vi "Modified Open URL in Default Browser core.vi"(4 "error in (no error)":errorcluster, 6 "Force IE? (F)":bool, 7 "url":string) -> (0 "error out":errorcluster, 3 "duplicate url":string)   [LabVIEW 2011]
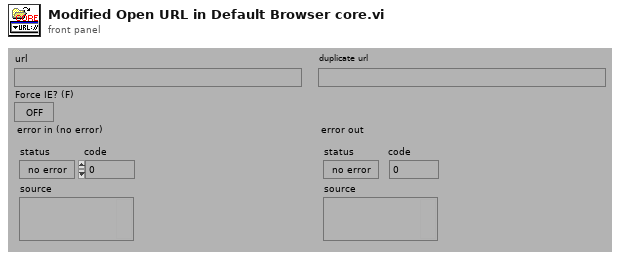
[diagram p1: front panel]
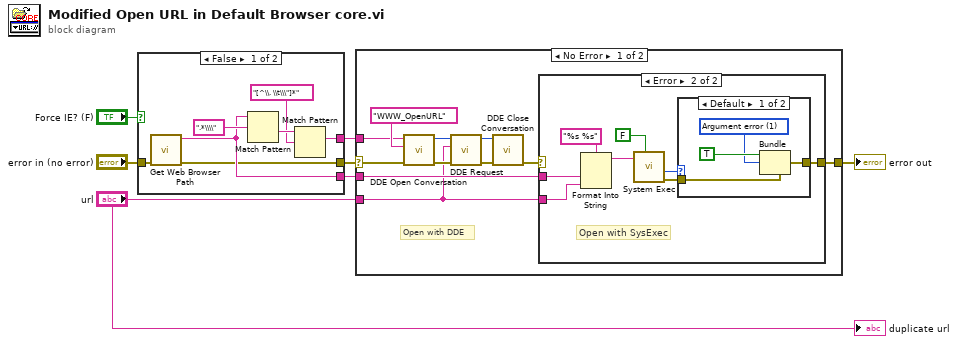
[diagram p0: block diagram]
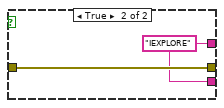
[diagram p2: hidden frame]
diagram:
  n1 = case shown="False" "Force IE? (F)" {
    tunnel: "error in (no error)" -> [w14 w16]
    tunnel: [w10 w15] -> w5
    tunnel: [w9 w15] -> w4
    tunnel: [w8 w16] -> w3
    frame False {
      n2 = call <vilib>:"Get Web Browser Path.vi"("error in (no error)"=w14) -> ("error out"=w8:errorcluster, "browser command"=w10:string)  [unwired: 5 out]
      n3 = Match Pattern(string=w10, regular expression=".*\\\\") -> (after substring=w12:string)  [unwired: 4 out]
      n4 = Match Pattern(string=w12, regular expression="[^\\. \\t\\\"]*") -> (match substring=w9:string)  [unwired: 4 out]
    }
    frame True {
      w15 = "IEXPLORE" ("regular expression")
    }
  }
  n5 = case shown="No Error" w3 {
    selector: w3 -> [w17 w42]
    tunnel: "url" -> [w18 _]
    tunnel: w4 -> [w22 _]
    tunnel: w5 -> [w21 _]
    tunnel: [w19 w42] -> w6
    frame No Error {
      # "Open with DDE"
      n6 = call <vilib>:"DDE Open Conversation.vi"("error in (no error)"=w17, "topic"="WWW_OpenURL", "service"=w22) -> ("error out"=w27:errorcluster, "conversation refnum"=w24:u32)  [unwired: 5 out]
      n7 = call <vilib>:"DDE Request.vi"("error in (no error)"=w27, "item"=w18, "conversation refnum in"=w24) -> ("error out"=w26:errorcluster, "conversation refnum out"=w25:u32)  [unwired: 5 out]
      n8 = call <vilib>:"DDE Close Conversation.vi"("error in (no error)"=w26, "conversation refnum"=w25) -> ("error out"=w20:errorcluster)  [unwired: 7 out]
      n9 = case shown="Error" w20 {
        selector: w20 -> [w28 _]
        tunnel: w21 -> [_ w35]
        tunnel: w18 -> [_ w34]
        tunnel: [w28 w29] -> w19
        frame No Error {
        }
        frame Error {
          # "Open with SysExec"
          n10 = Format Into String(format string="%s %s", w35, w34) -> (resulting string=w36:string)  [unwired: 2 in, 1 out]
          n11 = call <vilib>:"System Exec.vi"("wait until completion? (T)"=FALSE, "command line"=w36) -> ("error out"=w30:errorcluster, "return code"=w31:i32)  [unwired: 4 in, 4 out]
          n12 = case shown="Default" w31 {
            tunnel: w30 -> [w40 w41]
            tunnel: [w39 w41] -> w29
            frame Default {
              w37 = 1 items=["No error", "Argument error", "Memory is full", "Out of zone", "End of file", "File already open", "Generic file I/O error", "File not found", "File permission error", "Disk is full", "Duplicate path", "Too many files open", "System feature not enabled", "Resource file not found", "Cannot add resource", "Resource not found", "Image not found", "Image memory error", "Pen does not exist", "Config type invalid", "Config token not found", "Config parse error", "Config memory error", "Bad external code format", "Bad external code offset", "External code not present", "Null window", "Destroy window error", "Null menu", "Print aborted", "Bad print record", "Print driver error", "Windows error during printing", "Memory error during printing", "Print dialog error", "Generic print error", "Invalid device refnum", "Device not found", "Device parameter error", "Device unit error", "Cannot open device", "Device call aborted", "Generic error", "Cancelled by user", "Object ID too low", "Object ID too high", "Object not in heap", "Unknown heap", "Unknown object (invalid DefProc)", "Unknown object (DefProc not in table)", "Message out of range", "Invalid (null) method", "Unknown message", "Manager call not supported", "Bad address", "Network operation in progress", "Network operation timed out", "Connection is busy", "Network attribute not supported", "Network error", "Address in use", "System out of memory", "Connection aborted", "Connection refused", "Not connected", "Already connected", "Connection closed", "Initialization error (interapplication manager)", "Bad occurrence", "Wait on unbound occurrence handler", "Occurrence queue overflow", "Datalog type conflict", "Unused", "Unrecognized type (interapplication manager)", "Memory corrupt", "Failed to make temporary DLL", "Old CIN version", "Drag socket not found", "Failed to load drop-object", "Failed to register OLE object", "Failed to release OLE object", "Format specifier type mismatch", "Unknown format specifier", "Too few format specifiers", "Too many format specifiers", "Scan failed", "Newer CIN version", "Error converting to variant", "Runtime menu error", "Password tampered", "Variant attribute not found", "Incompatible variant data type", "Event data is not available", "Event Store is not present", "Occurrence is not found", "Event Queue is not created", "Event info is not available", "Refnum passed is NULL", "Error retrieving Class GUID", "Error retrieving CoClass GUID", "Error retrieving TypeLib GUID.", "Bad built application magic bytes.", "Specific driver is different from the specific driver associated with the Logical Name.", "There is no session opened to the class driver.", "Max Error", "MAX - Error with config objects", "MAX - Error loading configuration", "MAX - Group not supported"]
              n13 = Bundle(cluster=w40, "status"=TRUE, "code"=w37) -> (w39:errorcluster)  [unwired: 1 out]
            }
            frame 0 {
            }
          }
        }
      }
    }
    frame Error {
    }
  }
  "error out" <- w6
  "duplicate url" <- "url"
